vi "TimeTagToTimeStamp(Pair).vi"(10 "ttlw":u32 format="%.0x", 11 "tthw":u32 format="%.0x") -> (1 "IrigTime":T1, 2 "nSec counter":u64[](array[numeric]), 3 "time stamp":timestamp[](array[timestamp]))   [LabVIEW 2020, in "AIM664LV.lvlib"]
uses:
  AIM664LV.lvlib
  AFDX_Controls/IrigTime.ctl
panel:
  out "M":u32
  out "H":u32
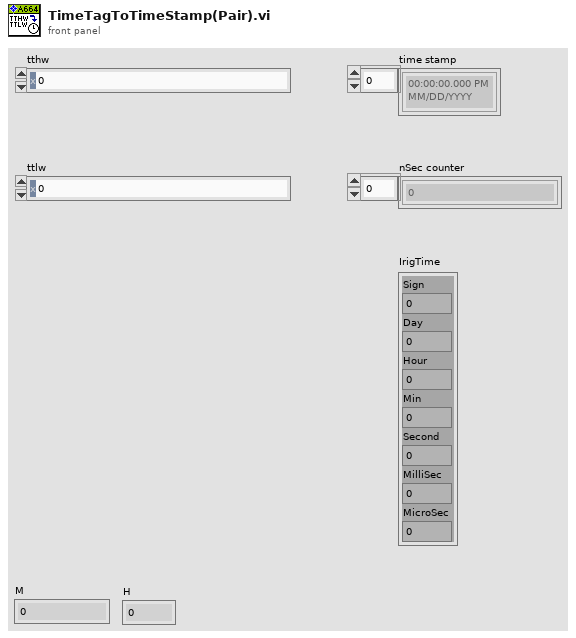
[diagram p1: front panel]
types:
  T1 = typedef "AIM664LV.lvlib/IrigTime.ctl" = cluster{"Sign":i32, "Day":u32, "Hour":u32, "Min":u32, "Second":u32, "MilliSec":u32, "MicroSec":u32}
  T2 = cluster{"Sign":i32, "Hour":u32, "Min":u32, "Second":u32, "Day":u32, "MilliSec":u32, "MicroSec":u32}
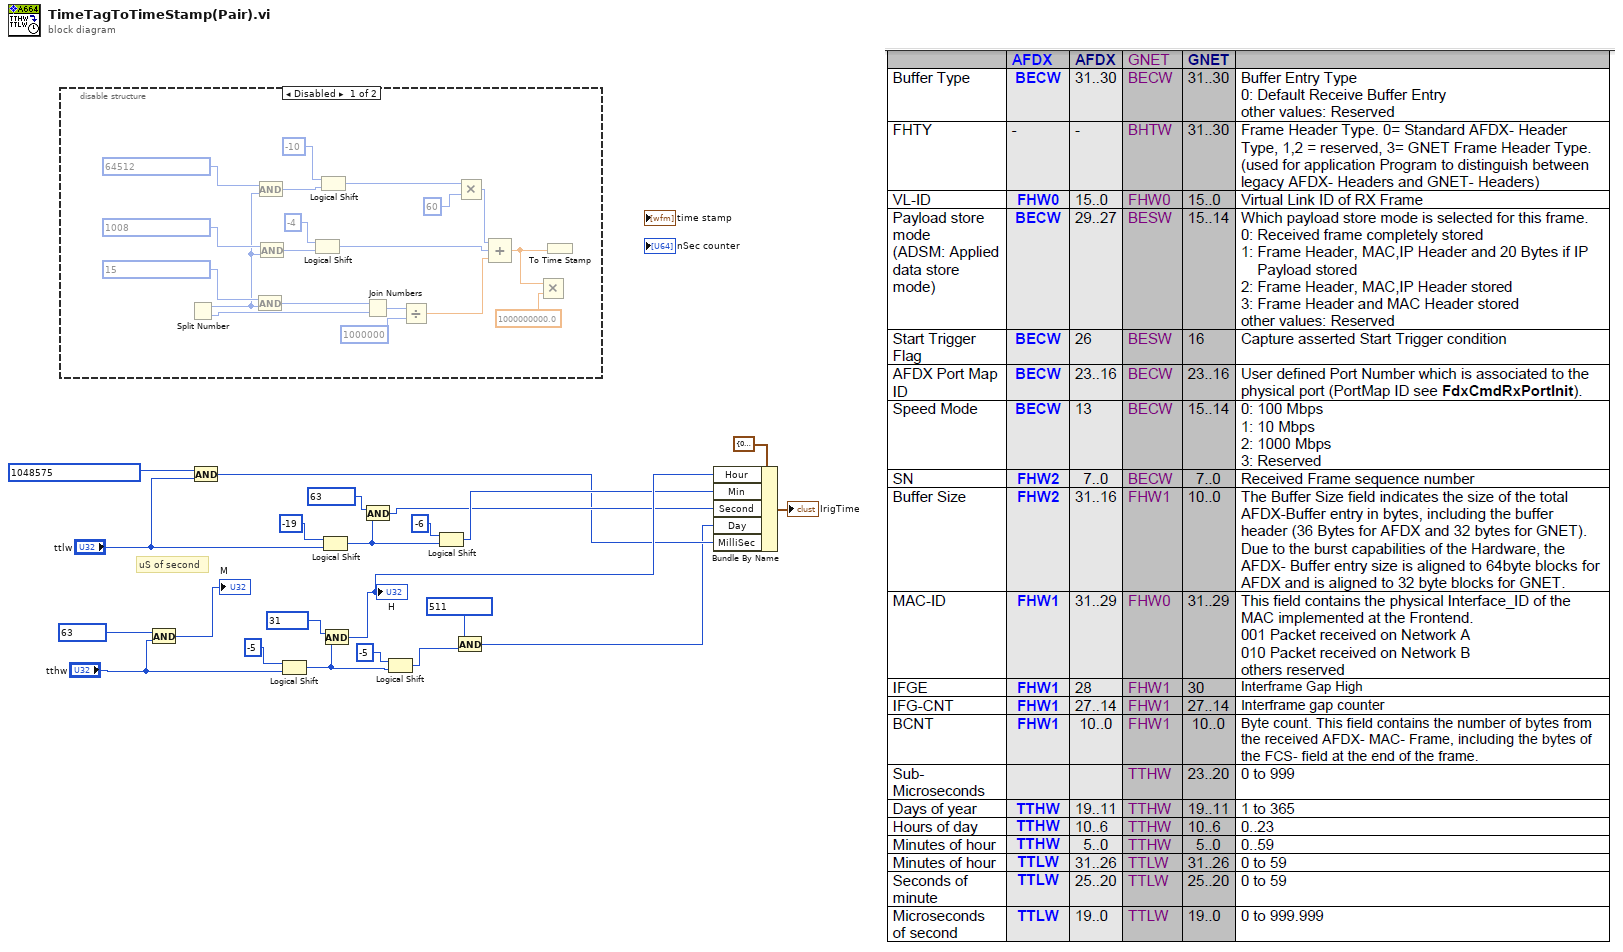
[diagram p0: block diagram]
diagram:
  # "uS of second"
  n1 = disable-structure shown="Disabled" {
    frame Disabled {
      n2 = Split Number() -> (hi(x)=w35:u16, lo(x)=w38:u16)  [unwired: 1 in]
      n3 = And(x=u16 15, y=w35) -> (x .and. y?=w39:u16)
      n4 = And(x=u16 64512, y=w35) -> (x .and. y?=w32:u16)
      n5 = And(x=u16 1008, y=w35) -> (x .and. y?=w34:u16)
      n6 = Logical Shift(y=i16 -4, x=w34) -> (x << y=w26:u16)
      n7 = Logical Shift(y=i16 -10, x=w32) -> (x << y=w30:u16)
      n8 = Join Numbers(hi=w39, lo=w38) -> ((hi.lo)=w25:u32)
      n9 = Divide(x=w25, y=u32 1000000) -> (x/y=w28:dbl)
      n10 = Multiply(x=w30, y=u16 60) -> (x*y=w27:u16)
      n11 = Compound Arithmetic op=ADD(w27, w26, w28) -> (w24:dbl)
      n12 = Multiply(x=w24, y=1000000000.0) -> ()  [unwired: 1 out]
      n13 = To Time Stamp(1:w24) -> ()  [unwired: 1 out]
    }
    frame Enabled {
    }
  }
  n14 = And(x=u32 63 ("Numeric"), y="tthw") -> (x .and. y?=→"M":u32)
  n15 = And(x=u32 1048575 ("Numeric"), y="ttlw") -> (x .and. y?=w2:u32)
  n16 = Logical Shift(y=i16 -5, x="tthw") -> (x << y=w15:u32)
  n17 = Logical Shift(y=i16 -19, x="ttlw") -> (x << y=w18:u32)
  n18 = And(x=u32 31 ("Numeric"), y=w15) -> (x .and. y?=w5:u32)
  "H" <- w5
  n19 = And(x=u32 63 ("Numeric"), y=w18) -> (x .and. y?=w3:u32)
  n20 = Logical Shift(y=i16 -5, x=w15) -> (x << y=w8:u32)
  n21 = Logical Shift(y=i16 -6, x=w18) -> (x << y=w4:u32)
  n22 = And(x=u32 511 ("Numeric"), y=w8) -> (x .and. y?=w1:u32)
  n23 = Bundle By Name(cluster=T2 {"Sign"=0, "Hour"=0, "Min"=0, "Second"=0, "Day"=0, "MilliSec"=0, "MicroSec"=0} ("IrigTime"), "Hour"=w5, "Min"=w4, "Second"=w3, "Day"=w1, "MilliSec"=w2) -> (→"IrigTime":T2)
